vi "生产调试用上位机.vi"() -> ()   [LabVIEW 2016]
uses:
  <vilib>/Utility/miscctls.llb/LVPointTypeDef.ctl
panel:
  in  "开机启动":bool
  in  "全屏":T1
  out "软件版本":string
  in  "报警查询":bool
  in  "日志查询":bool
  in  "主页按钮":bool
  in  "数据查询":bool
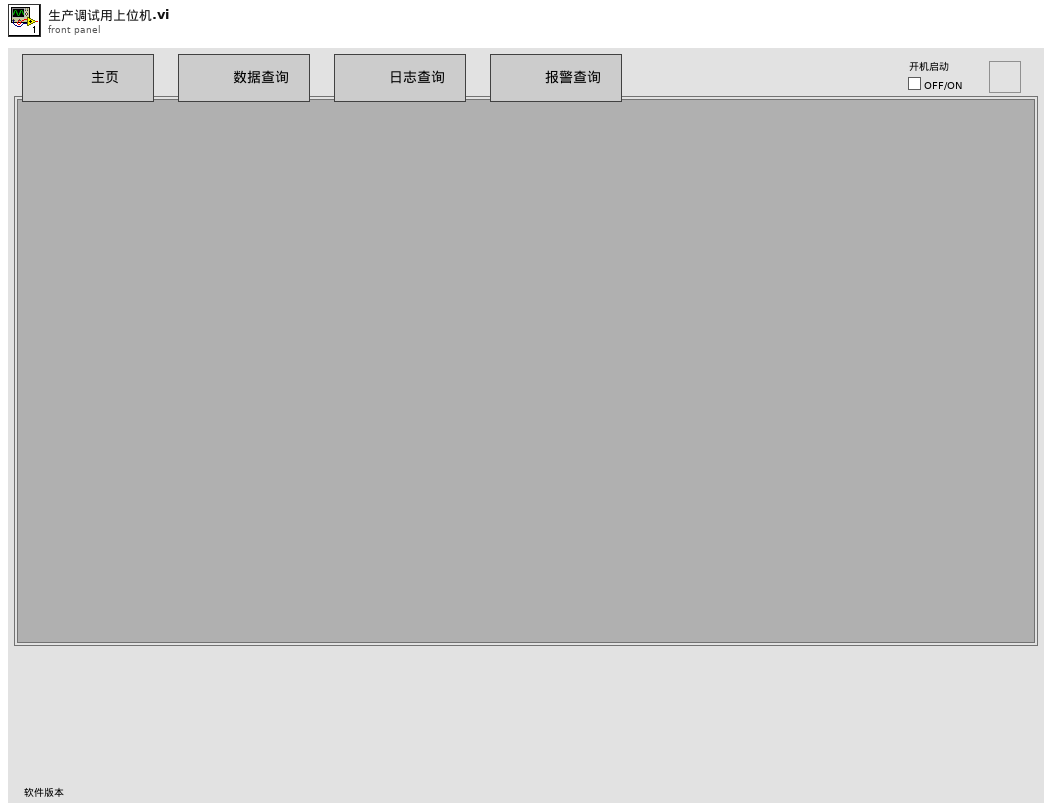
[diagram p1: front panel]
types:
  T1 = typedef "全屏按钮.ctl" = bool
  T2 = typedef "数据库类型.ctl" = enum16{"Access", "SQLite"}
  T3 = typedef "LVPointTypeDef.ctl" = cluster{"Horizontal":i16, "Vertical":i16}
  T4 = typedef "imagedata.ctl" = cluster{"image type":i32, "image depth":i32, "image":u8[], "mask":u8[], "colors":u32[], "Rectangle":cluster{"left":i16, "top":i16, "right":i16, "bottom":i16}}
  T5 = enum32{"Bad", "Idle", "Run top level", "Running"}
  T6 = typedef "数据查询.lvlib/数据查询单选控件.ctl" = enum32{"数据查询", "仪器数据", "仪器日志", "报警信息", "校准日志"}
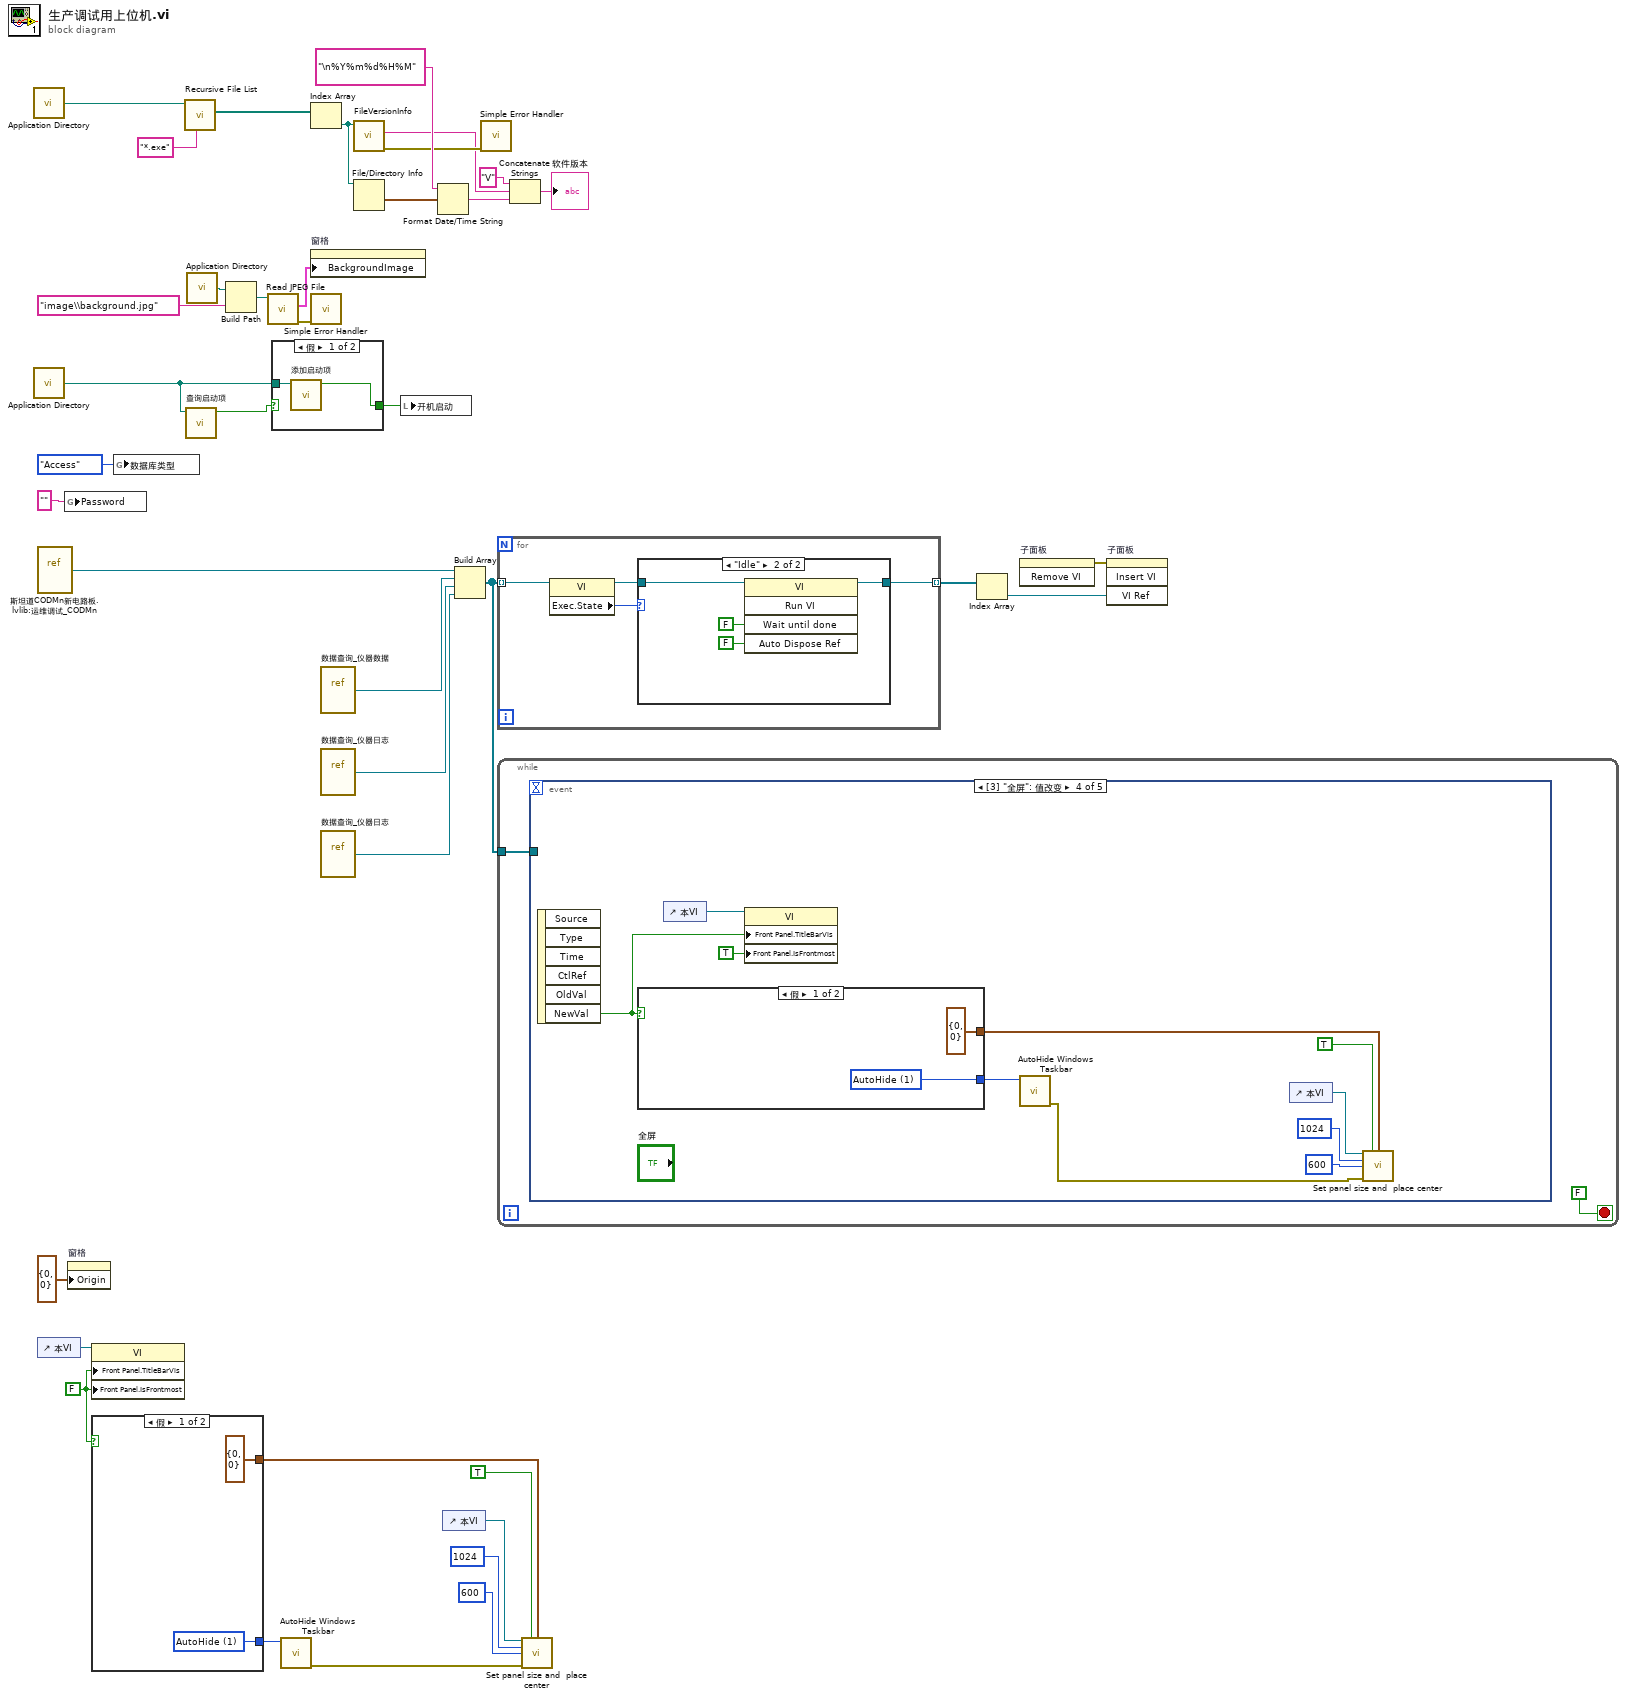
[diagram p0: block diagram]
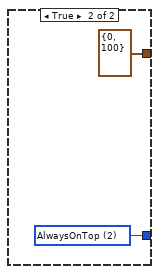
[diagram p2: hidden frame]
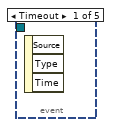
[diagram p5: hidden frame]
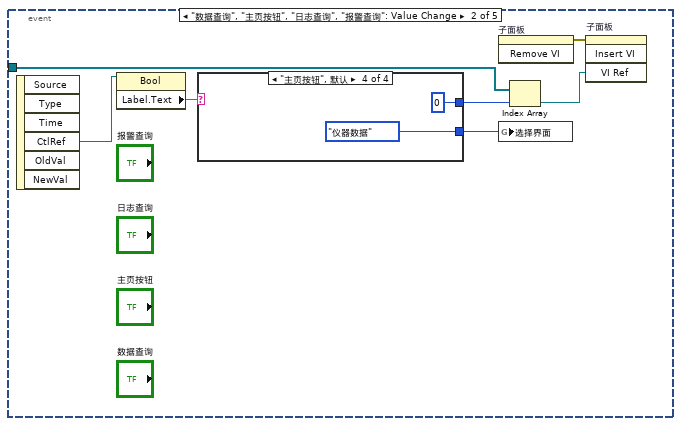
[diagram p6: hidden frame]
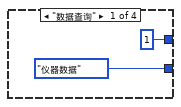
[diagram p7: hidden frame]
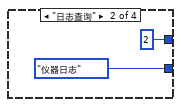
[diagram p8: hidden frame]
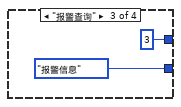
[diagram p9: hidden frame]
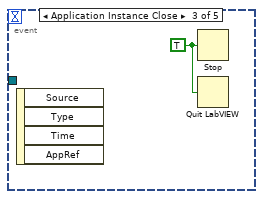
[diagram p10: hidden frame]
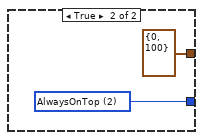
[diagram p11: hidden frame]
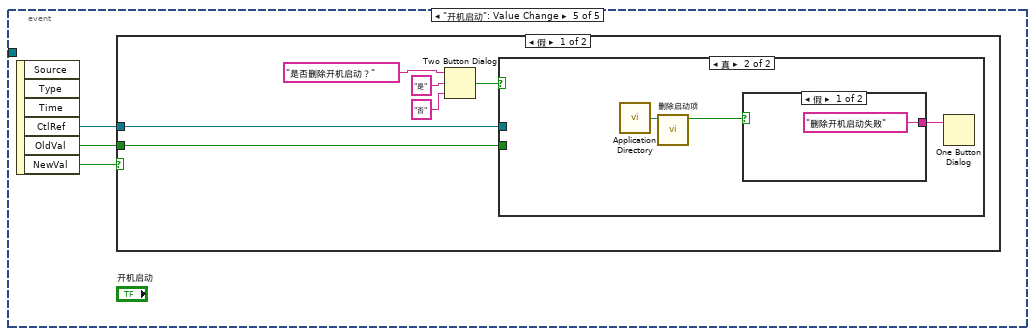
[diagram p12: hidden frame]
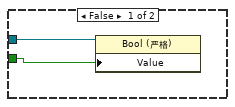
[diagram p13: hidden frame]
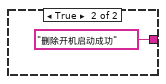
[diagram p14: hidden frame]
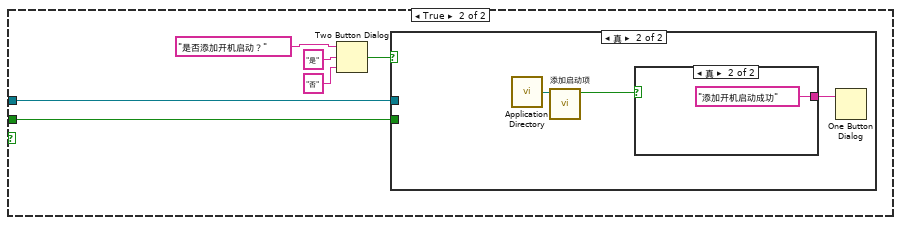
[diagram p15: hidden frame]
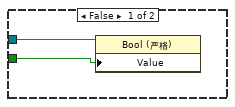
[diagram p16: hidden frame]
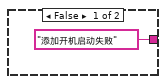
[diagram p17: hidden frame]
diagram:
  w1 = FALSE ("前面板窗口:在最前")
  n1 = call <vilib>:"Application Directory.vi"() -> ("Application Directory"=w32:path)
  n2 = call <vilib>:"Application Directory.vi"() -> ("Application Directory"=w12:path)
  n3 = vi-ref "斯坦道CODMn新电路板.lvlib:运维调试_CODMn.vi"() -> (w20:refnum<vi>)
  n4 = control-ref of="本VI"() -> (w2:refnum<vi>)
  n5 = global write "外部调用接口全局变量.vi" "Password"("" ("Password")) -> ()
  n6 = property on="窗格" class="Pane"("Origin"=T3 {"Horizontal"=0, "Vertical"=0} ("原点")) -> ()  [unwired: 2 in, 2 out]
  n7 = property class="VI"(reference=w2, "Front Panel.TitleBarVis"=w1, "Front Panel.IsFrontmost"=w1) -> ()  [unwired: 1 in, 2 out]
  n8 = case shown="假" w1 {
    tunnel: [w41 w43] -> w8
    tunnel: [cluster{"Horizontal":i16, "Vertical":i16} {"Horizontal"=0, "Vertical"=0} ("FP.WinOrigin in(H & V)") cluster{"Horizontal":i16, "Vertical":i16} {"Horizontal"=0, "Vertical"=100} ("FP.WinOrigin in(H & V)")] -> w9
    frame False {
      w41 = u8 1 items=["AutoHide"=1, "AlwaysOnTop"=2] ("Operation")
    }
    frame True {
      w43 = u8 2 items=["AutoHide"=1, "AlwaysOnTop"=2] ("Operation")
    }
  }
  n9 = global write "外部调用接口全局变量.vi" "数据库类型"(数据库类型."Access" ("数据库类型")) -> ()
  n10 = call <vilib>:"Recursive File List.vi"("pattern"="*.exe", "Folder Path"=w32) -> ("All Files in Dir"=w24:path[])  [unwired: 5 in, 4 out]
  n11 = call "查询启动项.vi"("启动文件路径"=w12) -> ("包含启动项"=w11:bool)  [unwired: 9 in, 1 out]
  n12 = call <vilib>:"Application Directory.vi"() -> ("Application Directory"=w39:path)
  n13 = Build Path(base path=w39, name or relative path="image\\background.jpg" ("名称或相对路径")) -> (appended path=w37:path)
  n14 = call <vilib>:"Read JPEG File.vi"("path to JPEG file"=w37) -> ("error out"=w35:errorcluster, "image data"=w36:T4)  [unwired: 8 in, 1 out]
  n15 = case shown="假" w11 {
    selector: w11 -> [_ w46]
    tunnel: w12 -> [w45 _]
    tunnel: [w44 w46] -> w10
    frame False {
      n16 = call "添加启动项.vi"("启动文件路径"=w45) -> ("添加成功标记"=w44:bool)  [unwired: 9 in, 1 out]
    }
    frame True {
    }
  }
  n17 = call "AutoHide Windows Taskbar.vi"("Operation"=w8) -> ("error out"=w7:errorcluster)  [unwired: 6 in]
  n18 = Index Array(array=w24) -> (element=w31:path)  [unwired: 1 in]
  n19 = property on="窗格" class="Pane"("BackgroundImage"=w36) -> ()  [unwired: 2 in, 2 out]
  n20 = call <vilib>:"Simple Error Handler.vi"("error in (no error)"=w35) -> ()  [unwired: 4 in, 5 out]
  n21 = vi-ref "数据查询_仪器数据.vi"() -> (w19:refnum<vi>)
  n22 = vi-ref "数据查询_仪器日志.vi"() -> (w13:refnum<vi>)
  n23 = vi-ref "数据查询_仪器日志.vi"() -> (w14:refnum<vi>)
  n24 = call <vilib>:"FileVersionInfo.vi"("Application Path in"=w31) -> ("error out"=w26:errorcluster, "File Version Info"=w25:string)  [unwired: 7 in, 2 out]
  n25 = File/Directory Info(path=w31) -> (last mod=w30:timestamp)  [unwired: 1 in, 6 out]
  n26 = local write "开机启动"(w10) -> ()
  n27 = Format Date/Time String(time format string (%c)="\n%Y%m%d%H%M" ("时间格式字符串(%c)"), seconds (now)=w30) -> (date/time string=w27:string)  [unwired: 1 in]
  n28 = control-ref of="本VI"() -> (w6:refnum<vi>)
  n29 = Build Array(w20, w19, w13, w14) -> (w15:refnum<vi>[])
  n30 = call <vilib>:"Simple Error Handler.vi"("error in (no error)"=w26) -> ()  [unwired: 4 in, 5 out]
  n31 = for {
    tunnel: [w48] -> w17 mode=indexing
    tunnel: w15 -> [w47] mode=indexing
    n32 = property class="VI"(reference=w47) -> (reference out=w49:refnum<vi>, "Exec.State"=w50:T5)  [unwired: 1 in, 1 out]
    n33 = case shown="\"Idle\"" w50 {
      tunnel: w49 -> [w51 w53]
      tunnel: [w51 w52] -> w48
      frame "Bad", Default {
      }
      frame "Idle" {
        n34 = invoke class="VI" method="Run VI"(reference=w53, "Wait until done"=FALSE ("结束前等待"), "Auto Dispose Ref"=FALSE ("自动销毁引用")) -> (reference out=w52:refnum<vi>)  [unwired: 2 in, 4 out]
      }
    }
  }
  n35 = while {
    tunnel: w15 -> [w56]
    stop <- FALSE stop-if-true
    n36 = event shown="[3] \"全屏\": 值改变" {
      selector: _ -> [_ _ _ _ _]
      dyn-events: _ -> [_ _ _ _ _]
      timeout: _ -> [_ _ _ _ _]
      tunnel: w56 -> [_ w62 _ _ _]
      event Timeout {
        n37 = event-data() -> ()  [unwired: 1 in, 3 out]
      }
      event "数据查询", "主页按钮", "日志查询", "报警查询": Value Change {
        n38 = event-data() -> ("CtlRef"=w61:refnum<vi>)  [unwired: 1 in, 5 out]
        n39 = property class="Bool"(reference=w61) -> ("Label.Text"=w60:string)  [unwired: 1 in, 2 out]
        n40 = case shown="\"主页按钮\", 默认" w60 {
          tunnel: [1 ("索引") 2 ("索引") 3 ("索引") 0 ("索引")] -> w59
          tunnel: [数据查询单选控件."仪器数据" ("选择界面") 数据查询单选控件."仪器日志" ("选择界面") 数据查询单选控件."报警信息" ("选择界面") 数据查询单选控件."仪器数据" ("选择界面")] -> w58
          frame "数据查询" {
          }
          frame "日志查询" {
          }
          frame "报警查询" {
          }
          frame "主页按钮", Default {
          }
        }
        n41 = invoke on="子面板" class="SubPnl" method="Remove VI"() -> (error out=w63:errorcluster)  [unwired: 3 in, 2 out]
        n42 = global write "全局变量.vi" "选择界面"(w58) -> ()
        n43 = Index Array(array=w62, index=w59) -> (element=w64:refnum<vi>)
        n44 = invoke on="子面板" class="SubPnl" method="Insert VI"(error in=w63, "VI Ref"=w64) -> ()  [unwired: 2 in, 4 out]
      }
      event Application Instance Close {
        w73 = TRUE ("停止？(T)")
        n45 = event-data() -> ()  [unwired: 1 in, 4 out]
        n46 = Stop(stop? (T)=w73) -> ()
        n47 = Quit LabVIEW(quit? (T)=w73) -> ()
      }
      event Value Change {
        n48 = event-data() -> ("NewVal"=w81:T1)  [unwired: 1 in, 5 out]
        n49 = case shown="假" w81 {
          tunnel: [w85 w87] -> w75
          tunnel: [cluster{"Horizontal":i16, "Vertical":i16} {"Horizontal"=0, "Vertical"=0} ("FP.WinOrigin in(H & V)") cluster{"Horizontal":i16, "Vertical":i16} {"Horizontal"=0, "Vertical"=100} ("FP.WinOrigin in(H & V)")] -> w74
          frame False {
            w85 = u8 1 items=["AutoHide"=1, "AlwaysOnTop"=2] ("Operation")
          }
          frame True {
            w87 = u8 2 items=["AutoHide"=1, "AlwaysOnTop"=2] ("Operation")
          }
        }
        n50 = control-ref of="本VI"() -> (w83:refnum<vi>)
        n51 = property class="VI"(reference=w83, "Front Panel.TitleBarVis"=w81, "Front Panel.IsFrontmost"=TRUE ("前面板窗口:在最前")) -> ()  [unwired: 1 in, 2 out]
        n52 = call "AutoHide Windows Taskbar.vi"("Operation"=w75) -> ("error out"=w76:errorcluster)  [unwired: 6 in]
        n53 = control-ref of="本VI"() -> (w77:refnum<vi>)
        n54 = call "Set panel size and  place center.vi"("VI引用句柄"=w77, "Close Reference (false)"=TRUE, "FP.WinOrigin in(H & V)"=w74, "Panel Width"=1024, "Panel Height"=600, "error in (no error)"=w76) -> ()  [unwired: 8 in, 2 out]
      }
      event "开机启动": Value Change {
        n55 = event-data() -> ("CtlRef"=w88:refnum<vi>, "OldVal"=w89:bool, "NewVal"=w90:bool)  [unwired: 1 in, 3 out]
        n56 = case shown="假" w90 {
          tunnel: w88 -> [w92 w105]
          tunnel: w89 -> [w91 w104]
          frame False {
            n57 = Two Button Dialog(message="是否删除开机启动？" ("消息"), 1:"否" ("F按钮名称（“取消”）"), 2:"是" ("T按钮名称（“确定”）")) -> (T button?=w93:bool)
            n58 = case shown="真" w93 {
              tunnel: w92 -> [w98 _]
              tunnel: w91 -> [w97 _]
              frame False {
                n59 = property class="Bool (严格)"(reference=w98, "Value"=w97) -> ()  [unwired: 1 in, 2 out]
              }
              frame True {
                n60 = call <vilib>:"Application Directory.vi"() -> ("Application Directory"=w100:path)
                n61 = call "删除启动项.vi"("启动文件路径"=w100) -> ("删除标记"=w99:bool)  [unwired: 9 in, 1 out]
                n62 = case shown="假" w99 {
                  tunnel: ["删除开机启动失败" ("T按钮名称（“确定”）") "删除开机启动成功" ("T按钮名称（“确定”）")] -> w101
                  frame False {
                  }
                  frame True {
                  }
                }
                n63 = One Button Dialog(message=w101) -> ()  [unwired: 1 in, 1 out]
              }
            }
          }
          frame True {
            n64 = Two Button Dialog(message="是否添加开机启动？" ("消息"), 1:"否" ("F按钮名称（“取消”）"), 2:"是" ("T按钮名称（“确定”）")) -> (T button?=w106:bool)
            n65 = case shown="真" w106 {
              tunnel: w105 -> [w111 _]
              tunnel: w104 -> [w110 _]
              frame False {
                n66 = property class="Bool (严格)"(reference=w111, "Value"=w110) -> ()  [unwired: 1 in, 2 out]
              }
              frame True {
                n67 = call <vilib>:"Application Directory.vi"() -> ("Application Directory"=w113:path)
                n68 = call "添加启动项.vi"("启动文件路径"=w113) -> ("添加成功标记"=w112:bool)  [unwired: 9 in, 1 out]
                n69 = case shown="真" w112 {
                  tunnel: ["添加开机启动失败" ("T按钮名称（“确定”）") "添加开机启动成功" ("T按钮名称（“确定”）")] -> w114
                  frame False {
                  }
                  frame True {
                  }
                }
                n70 = One Button Dialog(message=w114) -> ()  [unwired: 1 in, 1 out]
              }
            }
          }
        }
      }
    }
  }
  n71 = Concatenate Strings("V" ("字符串"), w25, w27) -> (→"软件版本":string)
  n72 = call "Set panel size and  place center.vi"("VI引用句柄"=w6, "Close Reference (false)"=TRUE, "FP.WinOrigin in(H & V)"=w9, "Panel Width"=1024, "Panel Height"=600, "error in (no error)"=w7) -> ()  [unwired: 8 in, 2 out]
  n73 = Index Array(array=w17) -> (element=w16:refnum<vi>)  [unwired: 1 in]
  n74 = invoke on="子面板" class="SubPnl" method="Remove VI"() -> (error out=w18:errorcluster)  [unwired: 3 in, 2 out]
  n75 = invoke on="子面板" class="SubPnl" method="Insert VI"(error in=w18, "VI Ref"=w16) -> ()  [unwired: 2 in, 4 out]
